vi "Smooth vertices by neighbours.vi"(10 "Smoothing rounds":i32=1, 11 "Vertex data":T1) -> (3 "Vertex data smoothened":T1)   [LabVIEW 2015, in "Morph Cortical Surfaces.lvlib"]
doc: "Smooth vertices by taking an average of the vertex's neighbours' coordinates."
uses:
  Morph Cortical Surfaces.lvlib
  Vertex data control.ctl
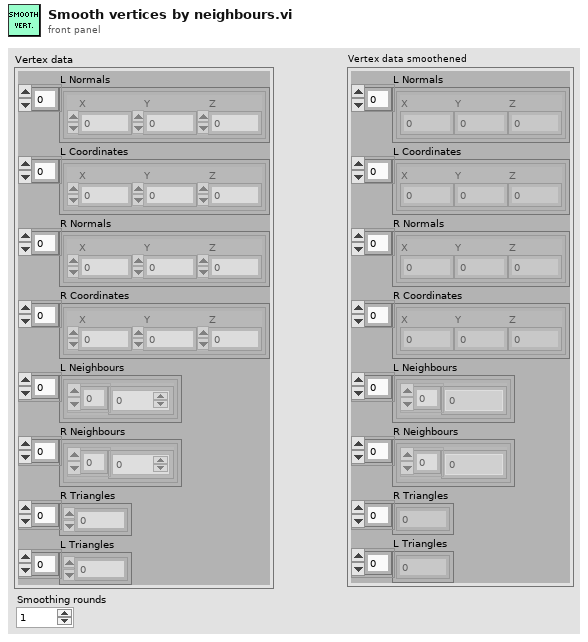
[diagram p1: front panel]
types:
  T1 = typedef "Morph Cortical Surfaces.lvlib/Vertex data control.ctl" = cluster{"L Normals":cluster{"X":sgl, "Y":sgl, "Z":sgl}[], "L Coordinates":cluster{"X":sgl, "Y":sgl, "Z":sgl}[], "R Normals":cluster{"X":sgl, "Y":sgl, "Z":sgl}[], "R Coordinates":cluster{"X":sgl, "Y":sgl, "Z":sgl}[], "L Neighbours":cluster{i32[]}[], "R Neighbours":cluster{i32[]}[], "R Triangles":i32[], "L Triangles":i32[]}
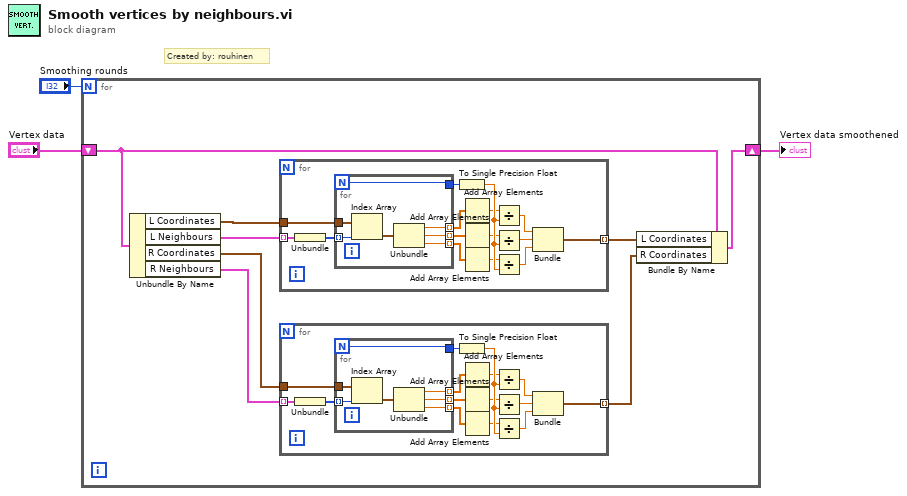
[diagram p0: block diagram]
diagram:
  # "Created by: rouhinen"
  n1 = for {
    N: "Smoothing rounds" -> [_]
    shift-right: [w11] -> w1
    shift-left: "Vertex data" -> [w9]
    n2 = Unbundle By Name(w9) -> ("L Coordinates"=w8:cluster{"X":sgl, "Y":sgl, "Z":sgl}[], "L Neighbours"=w7:cluster{i32[]}[], "R Coordinates"=w6:cluster{"X":sgl, "Y":sgl, "Z":sgl}[], "R Neighbours"=w5:cluster{i32[]}[])
    n3 = for {
      tunnel: w7 -> [w46] mode=indexing
      tunnel: w8 -> [w44]
      tunnel: [w34] -> w10 mode=indexing
      n4 = Unbundle(w46) -> (w45:i32[])
      n5 = for {
        N -> [w49]
        tunnel: w45 -> [w54] mode=indexing
        tunnel: w44 -> [w55]
        tunnel: [w52] -> w43 mode=indexing
        tunnel: [w51] -> w42 mode=indexing
        tunnel: [w50] -> w41 mode=indexing
        tunnel: [w49] -> w47
        n6 = Index Array(array=w55, index=w54) -> (element=w53:cluster{"X":sgl, "Y":sgl, "Z":sgl})
        n7 = Unbundle(w53) -> ("X"=w52:sgl, "Y"=w51:sgl, "Z"=w50:sgl)
      }
      n8 = To Single Precision Float(number=w47) -> (single precision float=w48:sgl)
      n9 = Add Array Elements(numeric array=w43) -> (sum=w40:sgl)
      n10 = Add Array Elements(numeric array=w42) -> (sum=w38:sgl)
      n11 = Add Array Elements(numeric array=w41) -> (sum=w39:sgl)
      n12 = Divide(x=w40, y=w48) -> (x/y=w36:sgl)
      n13 = Divide(x=w38, y=w48) -> (x/y=w37:sgl)
      n14 = Divide(x=w39, y=w48) -> (x/y=w35:sgl)
      n15 = Bundle(w36, w37, w35) -> (w34:cluster{sgl, sgl, sgl})  [unwired: 1 in]
    }
    n16 = for {
      tunnel: w5 -> [w24] mode=indexing
      tunnel: w6 -> [w22]
      tunnel: [w12] -> w4 mode=indexing
      n17 = Unbundle(w24) -> (w23:i32[])
      n18 = for {
        N -> [w27]
        tunnel: w23 -> [w32] mode=indexing
        tunnel: w22 -> [w33]
        tunnel: [w30] -> w21 mode=indexing
        tunnel: [w29] -> w20 mode=indexing
        tunnel: [w28] -> w19 mode=indexing
        tunnel: [w27] -> w25
        n19 = Index Array(array=w33, index=w32) -> (element=w31:cluster{"X":sgl, "Y":sgl, "Z":sgl})
        n20 = Unbundle(w31) -> ("X"=w30:sgl, "Y"=w29:sgl, "Z"=w28:sgl)
      }
      n21 = To Single Precision Float(number=w25) -> (single precision float=w26:sgl)
      n22 = Add Array Elements(numeric array=w21) -> (sum=w18:sgl)
      n23 = Add Array Elements(numeric array=w20) -> (sum=w16:sgl)
      n24 = Add Array Elements(numeric array=w19) -> (sum=w17:sgl)
      n25 = Divide(x=w18, y=w26) -> (x/y=w14:sgl)
      n26 = Divide(x=w16, y=w26) -> (x/y=w15:sgl)
      n27 = Divide(x=w17, y=w26) -> (x/y=w13:sgl)
      n28 = Bundle(w14, w15, w13) -> (w12:cluster{sgl, sgl, sgl})  [unwired: 1 in]
    }
    n29 = Bundle By Name(cluster=w9, "L Coordinates"=w10, "R Coordinates"=w4) -> (w11:T1)
  }
  "Vertex data smoothened" <- w1
